vi "cam1 analyse.vi"() -> (0 "W3&color":string)   [LabVIEW 2019]
uses:
  <vilib>/vision/Classification.llb/IMAQ Classifier Read Options.ctl
  <vilib>/vision/NI_Vision_Development_Module.lvlib
panel:
  out "R9 chiffre":string
  out "R8 chiffre":string
  out "R6 chiffre":string
  out "R3 chiffre":string
  out "B9 chiffre":string
  out "B8 chiffre":string
  out "B7 chiffre":string
  out "B6 chiffre":string
  out "B4 chiffre":string
  out "B3 chiffre":string
  out "B2 chiffre":string
  out "B1 chiffre":string
  out "W4 chiffre":string
  out "W6 chiffre":string
  out "W1 chiffre":string
  out "W2 chiffre":string
  out "W3 chiffre":string
  in  "R9":T1={"Global Rectangle"=[0, 0, 1279, 959], "Contours"=[{"ID"=enum."External", "Type"=3, "Coordinates"=[0, 0, 1279, 959]}]} {"Contours"."Type" items=["No Selection", "Point", "Line", "Rectangle", "Oval", "Polygon", "Freehand Region", "Annulus", "Unused2", "Unused3", "Broken Line", "Freehand Line", "Rotated Rectangle"]}
  out "R9":string[](array[string])
  in  "R8":T1={"Global Rectangle"=[0, 0, 1279, 959], "Contours"=[{"ID"=enum."External", "Type"=3, "Coordinates"=[0, 0, 1279, 959]}]} {"Contours"."Type" items=["No Selection", "Point", "Line", "Rectangle", "Oval", "Polygon", "Freehand Region", "Annulus", "Unused2", "Unused3", "Broken Line", "Freehand Line", "Rotated Rectangle"]}
  out "R8":string[](array[string])
  in  "R6":T1={"Global Rectangle"=[0, 0, 1279, 959], "Contours"=[{"ID"=enum."External", "Type"=3, "Coordinates"=[0, 0, 1279, 959]}]} {"Contours"."Type" items=["No Selection", "Point", "Line", "Rectangle", "Oval", "Polygon", "Freehand Region", "Annulus", "Unused2", "Unused3", "Broken Line", "Freehand Line", "Rotated Rectangle"]}
  out "R6":string[](array[string])
  in  "R3":T1={"Global Rectangle"=[0, 0, 1279, 959], "Contours"=[{"ID"=enum."External", "Type"=3, "Coordinates"=[0, 0, 1279, 959]}]} {"Contours"."Type" items=["No Selection", "Point", "Line", "Rectangle", "Oval", "Polygon", "Freehand Region", "Annulus", "Unused2", "Unused3", "Broken Line", "Freehand Line", "Rotated Rectangle"]}
  out "R3":string[](array[string])
  in  "B9":T1={"Global Rectangle"=[0, 0, 1279, 959], "Contours"=[{"ID"=enum."External", "Type"=3, "Coordinates"=[0, 0, 1279, 959]}]} {"Contours"."Type" items=["No Selection", "Point", "Line", "Rectangle", "Oval", "Polygon", "Freehand Region", "Annulus", "Unused2", "Unused3", "Broken Line", "Freehand Line", "Rotated Rectangle"]}
  out "B9":string[](array[string])
  in  "B8":T1={"Global Rectangle"=[0, 0, 1279, 959], "Contours"=[{"ID"=enum."External", "Type"=3, "Coordinates"=[0, 0, 1279, 959]}]} {"Contours"."Type" items=["No Selection", "Point", "Line", "Rectangle", "Oval", "Polygon", "Freehand Region", "Annulus", "Unused2", "Unused3", "Broken Line", "Freehand Line", "Rotated Rectangle"]}
  out "B8":string[](array[string])
  in  "B7":T1={"Global Rectangle"=[0, 0, 1279, 959], "Contours"=[{"ID"=enum."External", "Type"=3, "Coordinates"=[0, 0, 1279, 959]}]} {"Contours"."Type" items=["No Selection", "Point", "Line", "Rectangle", "Oval", "Polygon", "Freehand Region", "Annulus", "Unused2", "Unused3", "Broken Line", "Freehand Line", "Rotated Rectangle"]}
  out "B7":string[](array[string])
  in  "B6":T1={"Global Rectangle"=[0, 0, 1279, 959], "Contours"=[{"ID"=enum."External", "Type"=3, "Coordinates"=[0, 0, 1279, 959]}]} {"Contours"."Type" items=["No Selection", "Point", "Line", "Rectangle", "Oval", "Polygon", "Freehand Region", "Annulus", "Unused2", "Unused3", "Broken Line", "Freehand Line", "Rotated Rectangle"]}
  out "B6":string[](array[string])
  in  "B4":T1={"Global Rectangle"=[0, 0, 1279, 959], "Contours"=[{"ID"=enum."External", "Type"=3, "Coordinates"=[0, 0, 1279, 959]}]} {"Contours"."Type" items=["No Selection", "Point", "Line", "Rectangle", "Oval", "Polygon", "Freehand Region", "Annulus", "Unused2", "Unused3", "Broken Line", "Freehand Line", "Rotated Rectangle"]}
  out "B4":string[](array[string])
  in  "B3":T1={"Global Rectangle"=[0, 0, 1279, 959], "Contours"=[{"ID"=enum."External", "Type"=3, "Coordinates"=[0, 0, 1279, 959]}]} {"Contours"."Type" items=["No Selection", "Point", "Line", "Rectangle", "Oval", "Polygon", "Freehand Region", "Annulus", "Unused2", "Unused3", "Broken Line", "Freehand Line", "Rotated Rectangle"]}
  out "B3":string[](array[string])
  in  "B2":T1={"Global Rectangle"=[0, 0, 1279, 959], "Contours"=[{"ID"=enum."External", "Type"=3, "Coordinates"=[0, 0, 1279, 959]}]} {"Contours"."Type" items=["No Selection", "Point", "Line", "Rectangle", "Oval", "Polygon", "Freehand Region", "Annulus", "Unused2", "Unused3", "Broken Line", "Freehand Line", "Rotated Rectangle"]}
  out "B2":string[](array[string])
  in  "B1":T1={"Global Rectangle"=[0, 0, 1279, 959], "Contours"=[{"ID"=enum."External", "Type"=3, "Coordinates"=[0, 0, 1279, 959]}]} {"Contours"."Type" items=["No Selection", "Point", "Line", "Rectangle", "Oval", "Polygon", "Freehand Region", "Annulus", "Unused2", "Unused3", "Broken Line", "Freehand Line", "Rotated Rectangle"]}
  out "B1":string[](array[string])
  in  "W4":T1={"Global Rectangle"=[0, 0, 1279, 959], "Contours"=[{"ID"=enum."External", "Type"=3, "Coordinates"=[0, 0, 1279, 959]}]} {"Contours"."Type" items=["No Selection", "Point", "Line", "Rectangle", "Oval", "Polygon", "Freehand Region", "Annulus", "Unused2", "Unused3", "Broken Line", "Freehand Line", "Rotated Rectangle"]}
  out "W4":string[](array[string])
  in  "W6":T1={"Global Rectangle"=[0, 0, 1279, 959], "Contours"=[{"ID"=enum."External", "Type"=3, "Coordinates"=[0, 0, 1279, 959]}]} {"Contours"."Type" items=["No Selection", "Point", "Line", "Rectangle", "Oval", "Polygon", "Freehand Region", "Annulus", "Unused2", "Unused3", "Broken Line", "Freehand Line", "Rotated Rectangle"]}
  out "W6":string[](array[string])
  in  "W1":T1={"Global Rectangle"=[0, 0, 1279, 959], "Contours"=[{"ID"=enum."External", "Type"=3, "Coordinates"=[0, 0, 1279, 959]}]} {"Contours"."Type" items=["No Selection", "Point", "Line", "Rectangle", "Oval", "Polygon", "Freehand Region", "Annulus", "Unused2", "Unused3", "Broken Line", "Freehand Line", "Rotated Rectangle"]}
  out "W1":string[](array[string])
  out "W2":errorcluster
  in  "W2":T1={"Global Rectangle"=[0, 0, 1279, 959], "Contours"=[{"ID"=enum."External", "Type"=3, "Coordinates"=[0, 0, 1279, 959]}]} {"Contours"."Type" items=["No Selection", "Point", "Line", "Rectangle", "Oval", "Polygon", "Freehand Region", "Annulus", "Unused2", "Unused3", "Broken Line", "Freehand Line", "Rotated Rectangle"]}
  out "W2":string[](array[string])
  out "Coordinates":i32[](array[numeric])
  in  "W3":T1={"Global Rectangle"=[0, 0, 1279, 959], "Contours"=[{"ID"=enum."External", "Type"=3, "Coordinates"=[0, 0, 1279, 959]}]} {"Contours"."Type" items=["No Selection", "Point", "Line", "Rectangle", "Oval", "Polygon", "Freehand Region", "Annulus", "Unused2", "Unused3", "Broken Line", "Freehand Line", "Rotated Rectangle"]}
  out "Image Out":T2(plugin-control)
  out "W3":errorcluster
  out "W3":string[](array[string])
  in  "error in":errorcluster
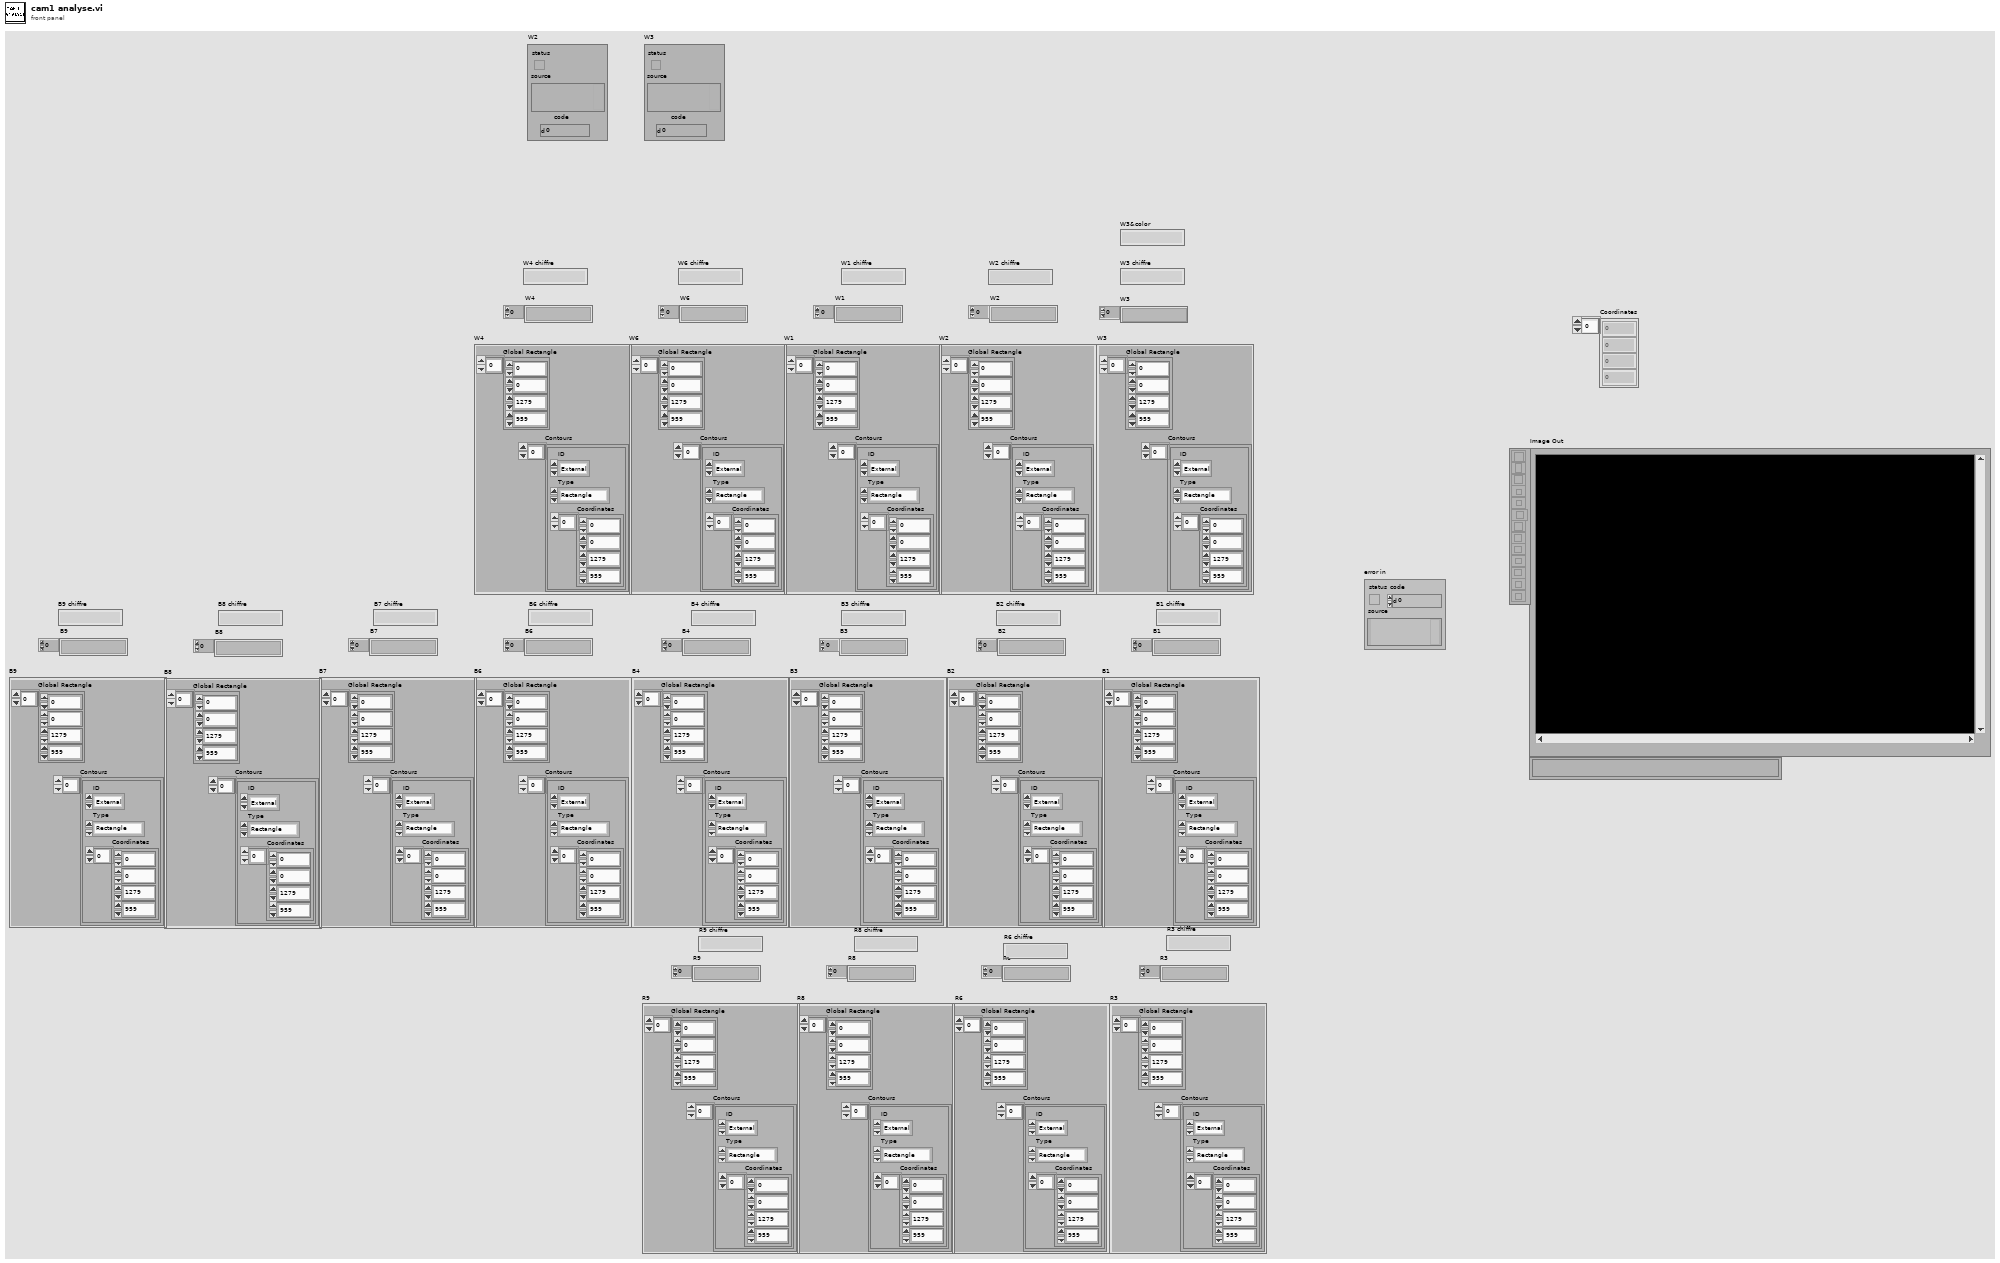
[diagram p1: front panel]
types:
  T1 = cluster{"Global Rectangle":i32[], "Contours":cluster{"ID":enum32{"External", "Internal"}, "Type":u32, "Coordinates":i32[]}[]}
  T2 = typedef "IMAQ Image.ctl" = refnum<image>
  T3 = typedef "IMAQ Classifier Read Options.ctl" = i32
  T4 = typedef "IMAQ Classifier Session.ctl" = refnum<k1>
  T5 = typedef "ROI Descriptor" = cluster{"Global Rectangle":i32[], "Contours":cluster{"ID":enum32{"External", "Internal"}, "Type":u32, "Coordinates":i32[]}[]}
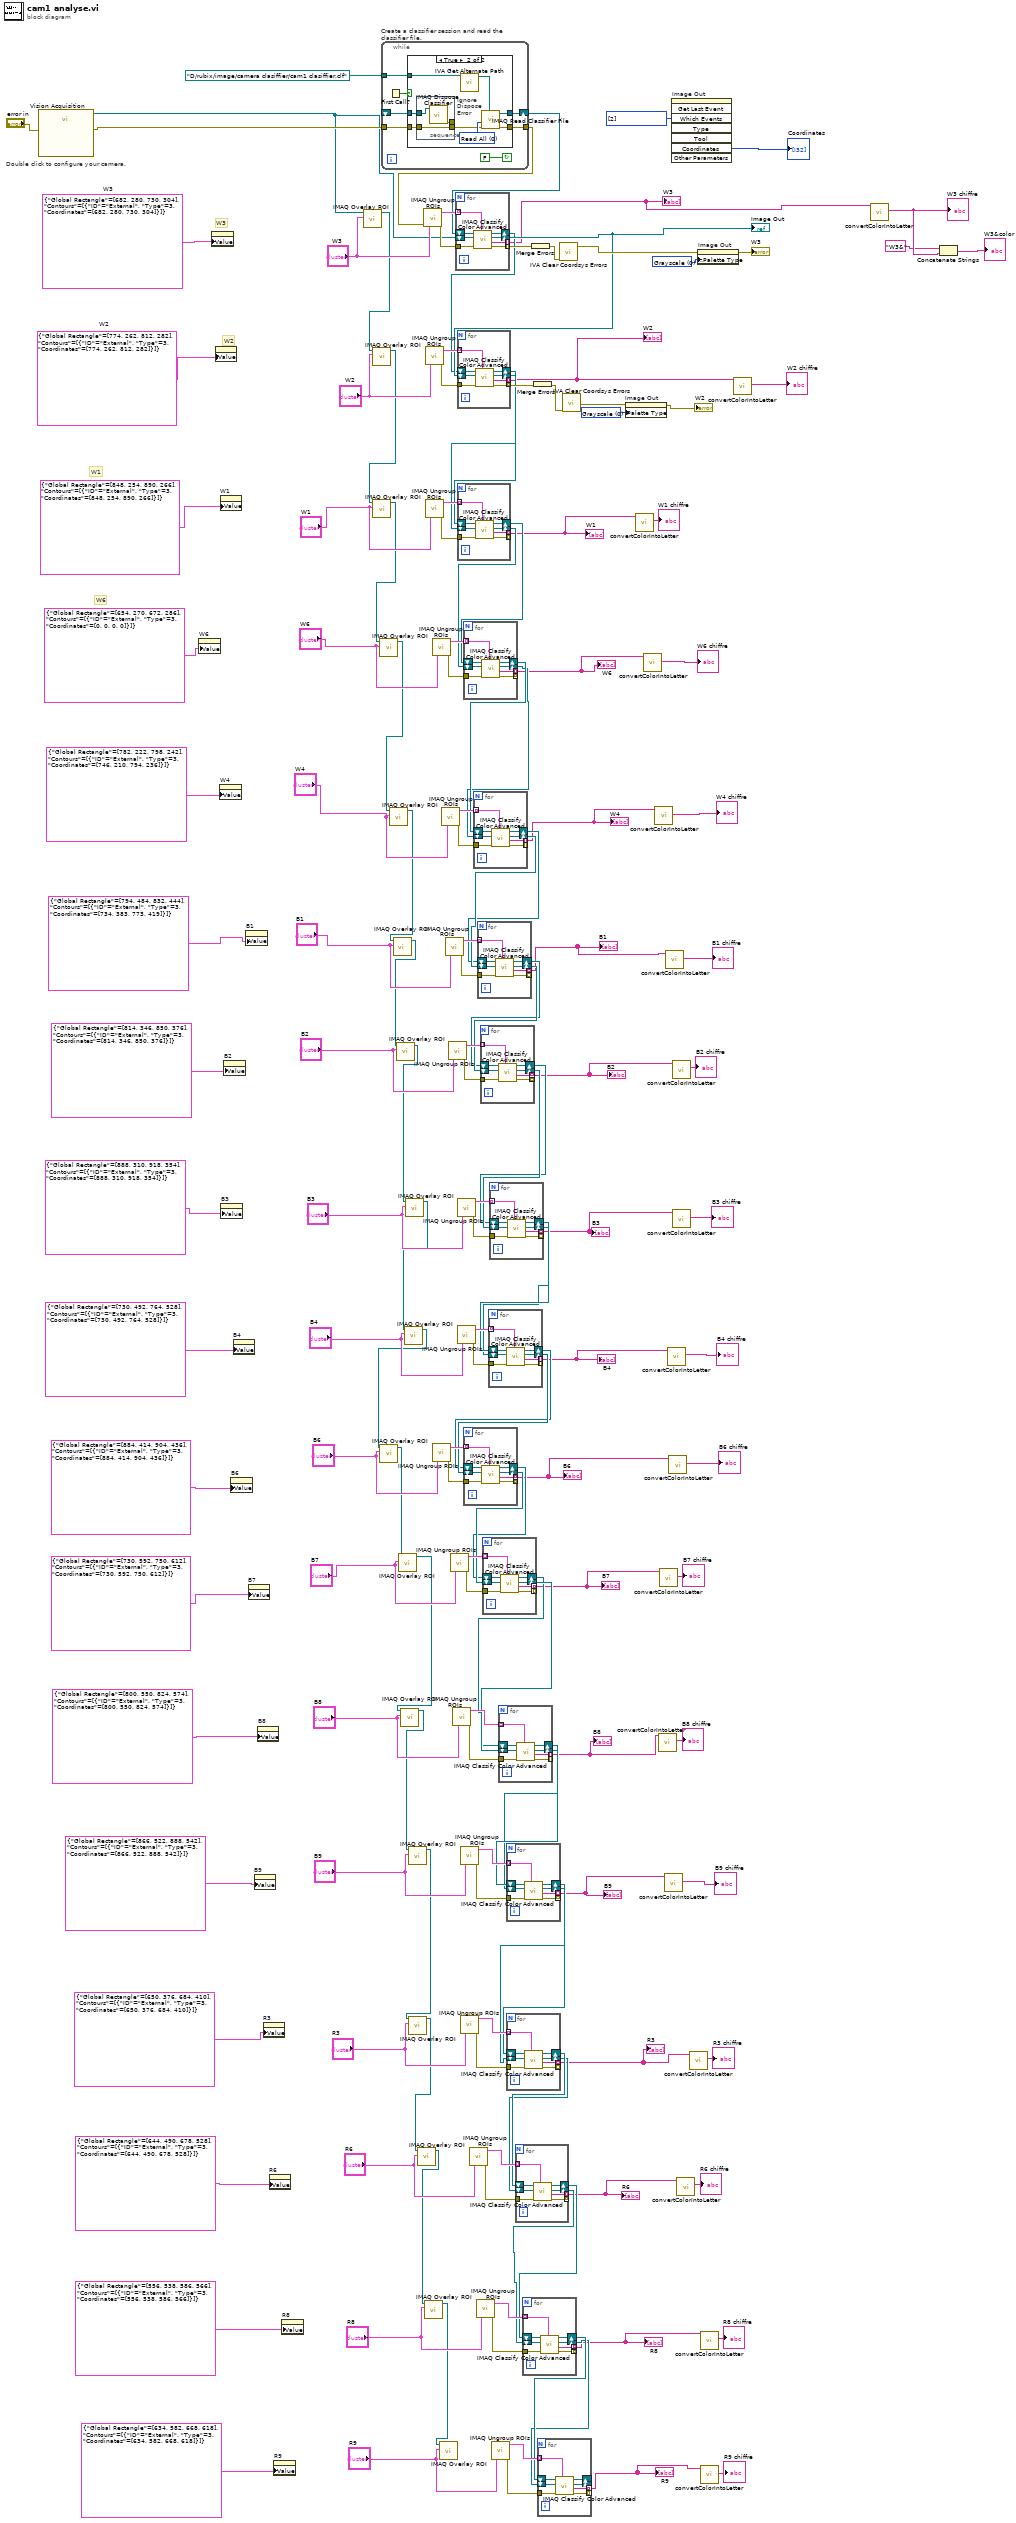
[diagram p0: block diagram]
diagram:
  w148 = u32 0 items=["Grayscale", "Binary", "Gradient", "Rainbow", "Temperature", "User Defined", "Binary 16 Bit", "Gradient 16 Bit", "Rainbow 16 Bit", "Temperature 16 Bit", "User Defined 16 Bit"] ("Palette:Palette Type")
  w158 = i32[] [2] items=["No Event"=0, "Click Event"=1, "Draw Event"=2, "Size Event"=4, "Scroll Event"=5, "Double Click Event"=8] ("Which Events")
  w159 = u32 0 items=["Grayscale", "Binary", "Gradient", "Rainbow", "Temperature", "User Defined", "Binary 16 Bit", "Gradient 16 Bit", "Rainbow 16 Bit", "Temperature 16 Bit", "User Defined 16 Bit"] ("Palette Type")
  # "W3"
  # "W2"
  # "W6"
  # "W1"
  # "Double click to configure your camera."
  n1 = call "Vision Acquisition"("error in"="error in") -> ("Image Out"=w144:T2, "error out"=w169:errorcluster)  [unwired: 24 in, 1 out]
  n2 = property on="W6" class="Clust (strict)"("Value"=T1 {"Global Rectangle"=[654, 270, 672, 286], "Contours"=[{"ID"=enum."External", "Type"=3, "Coordinates"=[0, 0, 0, 0]}]} ("ROI Descriptor (Color Classification 1)")) -> ()  [unwired: 2 in, 2 out]
  n3 = property on="W3" class="Clust (strict)"("Value"=T1 {"Global Rectangle"=[682, 280, 730, 304], "Contours"=[{"ID"=enum."External", "Type"=3, "Coordinates"=[682, 280, 730, 304]}]} ("ROI Descriptor (Color Classification 1)")) -> ()  [unwired: 2 in, 2 out]
  n4 = property on="W2" class="Clust (strict)"("Value"=T1 {"Global Rectangle"=[774, 262, 812, 282], "Contours"=[{"ID"=enum."External", "Type"=3, "Coordinates"=[774, 262, 812, 282]}]} ("ROI Descriptor (Color Classification 1)")) -> ()  [unwired: 2 in, 2 out]
  n5 = property on="W4" class="Clust (strict)"("Value"=T1 {"Global Rectangle"=[782, 222, 798, 242], "Contours"=[{"ID"=enum."External", "Type"=3, "Coordinates"=[746, 210, 794, 236]}]} ("ROI Descriptor (Color Classification 1)")) -> ()  [unwired: 2 in, 2 out]
  n6 = property on="W1" class="Clust (strict)"("Value"=T1 {"Global Rectangle"=[848, 254, 890, 266], "Contours"=[{"ID"=enum."External", "Type"=3, "Coordinates"=[848, 254, 890, 266]}]} ("ROI Descriptor (Color Classification 1)")) -> ()  [unwired: 2 in, 2 out]
  n7 = property on="B3" class="Clust (strict)"("Value"=T1 {"Global Rectangle"=[888, 310, 918, 354], "Contours"=[{"ID"=enum."External", "Type"=3, "Coordinates"=[888, 310, 918, 354]}]} ("ROI Descriptor (Color Classification 1)")) -> ()  [unwired: 2 in, 2 out]
  n8 = property on="B2" class="Clust (strict)"("Value"=T1 {"Global Rectangle"=[814, 346, 850, 376], "Contours"=[{"ID"=enum."External", "Type"=3, "Coordinates"=[814, 346, 850, 376]}]} ("ROI Descriptor (Color Classification 1)")) -> ()  [unwired: 2 in, 2 out]
  n9 = property on="B6" class="Clust (strict)"("Value"=T1 {"Global Rectangle"=[884, 414, 904, 436], "Contours"=[{"ID"=enum."External", "Type"=3, "Coordinates"=[884, 414, 904, 436]}]} ("ROI Descriptor (Color Classification 1)")) -> ()  [unwired: 2 in, 2 out]
  n10 = property on="B4" class="Clust (strict)"("Value"=T1 {"Global Rectangle"=[730, 492, 764, 528], "Contours"=[{"ID"=enum."External", "Type"=3, "Coordinates"=[730, 492, 764, 528]}]} ("ROI Descriptor (Color Classification 1)")) -> ()  [unwired: 2 in, 2 out]
  n11 = property on="B1" class="Clust (strict)"("Value"=T1 {"Global Rectangle"=[794, 484, 832, 444], "Contours"=[{"ID"=enum."External", "Type"=3, "Coordinates"=[734, 383, 773, 419]}]} ("ROI Descriptor (Color Classification 1)")) -> ()  [unwired: 2 in, 2 out]
  n12 = property on="B7" class="Clust (strict)"("Value"=T1 {"Global Rectangle"=[730, 592, 750, 612], "Contours"=[{"ID"=enum."External", "Type"=3, "Coordinates"=[730, 592, 750, 612]}]} ("ROI Descriptor (Color Classification 1)")) -> ()  [unwired: 2 in, 2 out]
  n13 = property on="B9" class="Clust (strict)"("Value"=T1 {"Global Rectangle"=[866, 522, 888, 542], "Contours"=[{"ID"=enum."External", "Type"=3, "Coordinates"=[866, 522, 888, 542]}]} ("ROI Descriptor (Color Classification 1)")) -> ()  [unwired: 2 in, 2 out]
  n14 = property on="B8" class="Clust (strict)"("Value"=T1 {"Global Rectangle"=[800, 550, 824, 574], "Contours"=[{"ID"=enum."External", "Type"=3, "Coordinates"=[800, 550, 824, 574]}]} ("ROI Descriptor (Color Classification 1)")) -> ()  [unwired: 2 in, 2 out]
  n15 = property on="R3" class="Clust (strict)"("Value"=T1 {"Global Rectangle"=[650, 376, 684, 410], "Contours"=[{"ID"=enum."External", "Type"=3, "Coordinates"=[650, 376, 684, 410]}]} ("ROI Descriptor (Color Classification 1)")) -> ()  [unwired: 2 in, 2 out]
  n16 = property on="R6" class="Clust (strict)"("Value"=T1 {"Global Rectangle"=[644, 490, 678, 528], "Contours"=[{"ID"=enum."External", "Type"=3, "Coordinates"=[644, 490, 678, 528]}]} ("ROI Descriptor (Color Classification 1)")) -> ()  [unwired: 2 in, 2 out]
  n17 = property on="R9" class="Clust (strict)"("Value"=T1 {"Global Rectangle"=[634, 582, 668, 618], "Contours"=[{"ID"=enum."External", "Type"=3, "Coordinates"=[634, 582, 668, 618]}]} ("ROI Descriptor (Color Classification 1)")) -> ()  [unwired: 2 in, 2 out]
  n18 = property on="R8" class="Clust (strict)"("Value"=T1 {"Global Rectangle"=[556, 538, 586, 566], "Contours"=[{"ID"=enum."External", "Type"=3, "Coordinates"=[556, 538, 586, 566]}]} ("ROI Descriptor (Color Classification 1)")) -> ()  [unwired: 2 in, 2 out]
  n19 = call "IMAQ Overlay ROI"("ROI Descriptor"="W3", "Image"=w144) -> ("Image Out"=w146:T2)  [unwired: 8 in, 1 out]
  n20 = call "IMAQ Overlay ROI"("ROI Descriptor"="W2", "Image"=w146) -> ("Image Out"=w139:T2)  [unwired: 8 in, 1 out]
  n21 = call "IMAQ Overlay ROI"("ROI Descriptor"="W1", "Image"=w139) -> ("Image Out"=w131:T2)  [unwired: 8 in, 1 out]
  n22 = call "IMAQ Overlay ROI"("ROI Descriptor"="W6", "Image"=w131) -> ("Image Out"=w123:T2)  [unwired: 8 in, 1 out]
  n23 = while "Create a classifier session and read the classifier file." {
    shift-right: [w177] -> w161
    shift-left: _ -> [w176]
    tunnel: w169 -> [w174]
    tunnel: [w173] -> w167
    tunnel: path "D:/rubix/image/camera clasiffier/cam1 clasiffier.clf" ("File Path") -> [w172]
    stop <- FALSE continue-if-true
    n24 = First Call?() -> (First Call?: T/F=w171:bool)
    n25 = case shown="True" w171 {
      tunnel: [w179 w186] -> w177
      tunnel: w176 -> [w179 w184]
      tunnel: w174 -> [w178 w183]
      tunnel: [w178 w185] -> w173
      tunnel: w172 -> [_ w181]
      frame False {
      }
      frame True {
        w187 = T3 0 items=["Read All", "Add Samples, Do Not Change Options", "Read Options, Do Not Add Samples"] ("Read Options")
        # "Ignore Dispose Error"
        n26 = stacked-sequence {
          tunnel: w184 -> [w190]
          tunnel: w183 -> [w189]
          tunnel: [w189] -> w182
          tunnel: [w188] -> _
          frame #0 {
            n27 = call "IMAQ Dispose Classifier"("Classifier Session"=w190) -> ("error out"=w188:errorcluster)  [unwired: 1 in, 9 out]
          }
        }
        n28 = call <vilib>:"IVA Get Alternate Path.vi"("Path In"=w181) -> ("Path Out"=w180:path)  [unwired: 10 out]
        n29 = call "IMAQ Read Classifier File"("File Path"=w180, "error in (no error)"=w182, "Read Options"=w187) -> ("error out"=w185:errorcluster, "Classifier Session"=w186:T4)  [unwired: 1 in, 6 out]
      }
    }
  }
  n30 = call "IMAQ Overlay ROI"("ROI Descriptor"="W4", "Image"=w123) -> ("Image Out"=w116:T2)  [unwired: 8 in, 1 out]
  n31 = call "IMAQ Overlay ROI"("ROI Descriptor"="B1", "Image"=w116) -> ("Image Out"=w111:T2)  [unwired: 8 in, 1 out]
  n32 = call "IMAQ Overlay ROI"("ROI Descriptor"="B2", "Image"=w111) -> ("Image Out"=w104:T2)  [unwired: 8 in, 1 out]
  n33 = call "IMAQ Overlay ROI"("ROI Descriptor"="B3", "Image"=w104) -> ("Image Out"=w94:T2)  [unwired: 8 in, 1 out]
  n34 = call "IMAQ Overlay ROI"("ROI Descriptor"="B4", "Image"=w94) -> ("Image Out"=w90:T2)  [unwired: 8 in, 1 out]
  n35 = call "IMAQ Overlay ROI"("ROI Descriptor"="B6", "Image"=w90) -> ("Image Out"=w81:T2)  [unwired: 8 in, 1 out]
  n36 = call "IMAQ Overlay ROI"("ROI Descriptor"="B7", "Image"=w81) -> ("Image Out"=w76:T2)  [unwired: 8 in, 1 out]
  n37 = call "IMAQ Overlay ROI"("ROI Descriptor"="B8", "Image"=w76) -> ("Image Out"=w69:T2)  [unwired: 8 in, 1 out]
  n38 = call "IMAQ Overlay ROI"("ROI Descriptor"="B9", "Image"=w69) -> ("Image Out"=w62:T2)  [unwired: 8 in, 1 out]
  n39 = call "IMAQ Overlay ROI"("ROI Descriptor"="R3", "Image"=w62) -> ("Image Out"=w55:T2)  [unwired: 8 in, 1 out]
  n40 = call "IMAQ Overlay ROI"("ROI Descriptor"="R6", "Image"=w55) -> ("Image Out"=w48:T2)  [unwired: 8 in, 1 out]
  n41 = call "IMAQ Ungroup ROIs"("error in (no error)"=w167, "ROI Descriptor"="W3") -> ("error out"=w166:errorcluster, "ROI Descriptors out"=w165:T5[])  [unwired: 2 out]
  n42 = call "IMAQ Overlay ROI"("ROI Descriptor"="R8", "Image"=w48) -> ("Image Out"=w41:T2)  [unwired: 8 in, 1 out]
  n43 = call "IMAQ Ungroup ROIs"("ROI Descriptor"="W2") -> ("error out"=w154:errorcluster, "ROI Descriptors out"=w153:T5[])  [unwired: 1 in, 2 out]
  n44 = call "IMAQ Ungroup ROIs"("ROI Descriptor"="W1") -> ("error out"=w141:errorcluster, "ROI Descriptors out"=w140:T5[])  [unwired: 1 in, 2 out]
  n45 = call "IMAQ Ungroup ROIs"("ROI Descriptor"="W6") -> ("error out"=w134:errorcluster, "ROI Descriptors out"=w133:T5[])  [unwired: 1 in, 2 out]
  n46 = call "IMAQ Ungroup ROIs"("ROI Descriptor"="B6") -> ("error out"=w93:errorcluster, "ROI Descriptors out"=w92:T5[])  [unwired: 1 in, 2 out]
  n47 = call "IMAQ Overlay ROI"("ROI Descriptor"="R9", "Image"=w41) -> ()  [unwired: 8 in, 2 out]
  n48 = call "IMAQ Ungroup ROIs"("ROI Descriptor"="W4") -> ("error out"=w127:errorcluster, "ROI Descriptors out"=w126:T5[])  [unwired: 1 in, 2 out]
  n49 = call "IMAQ Ungroup ROIs"("ROI Descriptor"="B1") -> ("error out"=w120:errorcluster, "ROI Descriptors out"=w119:T5[])  [unwired: 1 in, 2 out]
  n50 = call "IMAQ Ungroup ROIs"("ROI Descriptor"="B2") -> ("error out"=w114:errorcluster, "ROI Descriptors out"=w113:T5[])  [unwired: 1 in, 2 out]
  n51 = call "IMAQ Ungroup ROIs"("ROI Descriptor"="B7") -> ("error out"=w86:errorcluster, "ROI Descriptors out"=w85:T5[])  [unwired: 1 in, 2 out]
  n52 = call "IMAQ Ungroup ROIs"("ROI Descriptor"="B8") -> ("error out"=w79:errorcluster, "ROI Descriptors out"=w78:T5[])  [unwired: 1 in, 2 out]
  n53 = for {
    tunnel: [w198] -> w20 mode=indexing
    tunnel: [w197] -> w164 mode=indexing
    tunnel: w166 -> [w195]
    tunnel: w165 -> [w194] mode=indexing
    shift-right: [w192] -> w143
    shift-left: w144 -> [w193]
    shift-right: [w191] -> w142
    shift-left: w161 -> [w196]
    n54 = call "IMAQ Classify Color Advanced"("ROI Descriptor"=w194, "error in (no error)"=w195, "Image"=w193, "Classifier Session"=w196) -> ("error out"=w197:errorcluster, "Class"=w198:string, "Image (dup)"=w192:T2, "Classifier Session (dup)"=w191:T4)  [unwired: 4 out]
  }
  "W3" <- w20
  "Image Out" <- w143
  n55 = for {
    tunnel: [w206] -> w36 mode=indexing
    tunnel: [w205] -> w152 mode=indexing
    tunnel: w154 -> [w203]
    tunnel: w153 -> [w202] mode=indexing
    shift-right: [w200] -> w137
    shift-left: w143 -> [w201]
    shift-right: [w199] -> w138
    shift-left: w142 -> [w204]
    n56 = call "IMAQ Classify Color Advanced"("ROI Descriptor"=w202, "error in (no error)"=w203, "Image"=w201, "Classifier Session"=w204) -> ("error out"=w205:errorcluster, "Class"=w206:string, "Image (dup)"=w200:T2, "Classifier Session (dup)"=w199:T4)  [unwired: 4 out]
  }
  "W2" <- w36
  n57 = for {
    tunnel: [w214] -> w35 mode=indexing
    tunnel: [w213] -> _ mode=indexing
    tunnel: w141 -> [w211]
    tunnel: w140 -> [w210] mode=indexing
    shift-right: [w208] -> w130
    shift-left: w137 -> [w209]
    shift-right: [w207] -> w129
    shift-left: w138 -> [w212]
    n58 = call "IMAQ Classify Color Advanced"("ROI Descriptor"=w210, "error in (no error)"=w211, "Image"=w209, "Classifier Session"=w212) -> ("error out"=w213:errorcluster, "Class"=w214:string, "Image (dup)"=w208:T2, "Classifier Session (dup)"=w207:T4)  [unwired: 4 out]
  }
  "W1" <- w35
  n59 = call "IMAQ Ungroup ROIs"("ROI Descriptor"="B4") -> ("error out"=w100:errorcluster, "ROI Descriptors out"=w99:T5[])  [unwired: 1 in, 2 out]
  n60 = call "IMAQ Ungroup ROIs"("ROI Descriptor"="B3") -> ("error out"=w107:errorcluster, "ROI Descriptors out"=w106:T5[])  [unwired: 1 in, 2 out]
  n61 = call "IMAQ Ungroup ROIs"("ROI Descriptor"="B9") -> ("error out"=w72:errorcluster, "ROI Descriptors out"=w71:T5[])  [unwired: 1 in, 2 out]
  n62 = call "IMAQ Ungroup ROIs"("ROI Descriptor"="R3") -> ("error out"=w65:errorcluster, "ROI Descriptors out"=w64:T5[])  [unwired: 1 in, 2 out]
  n63 = for {
    tunnel: [w222] -> w34 mode=indexing
    tunnel: [w221] -> _ mode=indexing
    tunnel: w134 -> [w219]
    tunnel: w133 -> [w218] mode=indexing
    shift-right: [w216] -> w124
    shift-left: w130 -> [w217]
    shift-right: [w215] -> w125
    shift-left: w129 -> [w220]
    n64 = call "IMAQ Classify Color Advanced"("ROI Descriptor"=w218, "error in (no error)"=w219, "Image"=w217, "Classifier Session"=w220) -> ("error out"=w221:errorcluster, "Class"=w222:string, "Image (dup)"=w216:T2, "Classifier Session (dup)"=w215:T4)  [unwired: 4 out]
  }
  "W6" <- w34
  n65 = call "IMAQ Ungroup ROIs"("ROI Descriptor"="R6") -> ("error out"=w58:errorcluster, "ROI Descriptors out"=w57:T5[])  [unwired: 1 in, 2 out]
  n66 = for {
    tunnel: [w230] -> w33 mode=indexing
    tunnel: [w229] -> _ mode=indexing
    tunnel: w127 -> [w227]
    tunnel: w126 -> [w226] mode=indexing
    shift-right: [w224] -> w118
    shift-left: w124 -> [w225]
    shift-right: [w223] -> w117
    shift-left: w125 -> [w228]
    n67 = call "IMAQ Classify Color Advanced"("ROI Descriptor"=w226, "error in (no error)"=w227, "Image"=w225, "Classifier Session"=w228) -> ("error out"=w229:errorcluster, "Class"=w230:string, "Image (dup)"=w224:T2, "Classifier Session (dup)"=w223:T4)  [unwired: 4 out]
  }
  "W4" <- w33
  n68 = call "IMAQ Ungroup ROIs"("ROI Descriptor"="R8") -> ("error out"=w51:errorcluster, "ROI Descriptors out"=w50:T5[])  [unwired: 1 in, 2 out]
  n69 = for {
    tunnel: [w238] -> w32 mode=indexing
    tunnel: [w237] -> _ mode=indexing
    tunnel: w120 -> [w235]
    tunnel: w119 -> [w234] mode=indexing
    shift-right: [w232] -> w110
    shift-left: w118 -> [w233]
    shift-right: [w231] -> w109
    shift-left: w117 -> [w236]
    n70 = call "IMAQ Classify Color Advanced"("ROI Descriptor"=w234, "error in (no error)"=w235, "Image"=w233, "Classifier Session"=w236) -> ("error out"=w237:errorcluster, "Class"=w238:string, "Image (dup)"=w232:T2, "Classifier Session (dup)"=w231:T4)  [unwired: 4 out]
  }
  "B1" <- w32
  n71 = for {
    tunnel: [w246] -> w31 mode=indexing
    tunnel: [w245] -> _ mode=indexing
    tunnel: w114 -> [w243]
    tunnel: w113 -> [w242] mode=indexing
    shift-right: [w240] -> w103
    shift-left: w110 -> [w241]
    shift-right: [w239] -> w102
    shift-left: w109 -> [w244]
    n72 = call "IMAQ Classify Color Advanced"("ROI Descriptor"=w242, "error in (no error)"=w243, "Image"=w241, "Classifier Session"=w244) -> ("error out"=w245:errorcluster, "Class"=w246:string, "Image (dup)"=w240:T2, "Classifier Session (dup)"=w239:T4)  [unwired: 4 out]
  }
  "B2" <- w31
  n73 = for {
    tunnel: [w254] -> w30 mode=indexing
    tunnel: [w253] -> _ mode=indexing
    tunnel: w107 -> [w251]
    tunnel: w106 -> [w250] mode=indexing
    shift-right: [w248] -> w97
    shift-left: w103 -> [w249]
    shift-right: [w247] -> w98
    shift-left: w102 -> [w252]
    n74 = call "IMAQ Classify Color Advanced"("ROI Descriptor"=w250, "error in (no error)"=w251, "Image"=w249, "Classifier Session"=w252) -> ("error out"=w253:errorcluster, "Class"=w254:string, "Image (dup)"=w248:T2, "Classifier Session (dup)"=w247:T4)  [unwired: 4 out]
  }
  "B3" <- w30
  n75 = for {
    tunnel: [w262] -> w29 mode=indexing
    tunnel: [w261] -> _ mode=indexing
    tunnel: w100 -> [w259]
    tunnel: w99 -> [w258] mode=indexing
    shift-right: [w256] -> w89
    shift-left: w97 -> [w257]
    shift-right: [w255] -> w88
    shift-left: w98 -> [w260]
    n76 = call "IMAQ Classify Color Advanced"("ROI Descriptor"=w258, "error in (no error)"=w259, "Image"=w257, "Classifier Session"=w260) -> ("error out"=w261:errorcluster, "Class"=w262:string, "Image (dup)"=w256:T2, "Classifier Session (dup)"=w255:T4)  [unwired: 4 out]
  }
  "B4" <- w29
  n77 = for {
    tunnel: [w270] -> w28 mode=indexing
    tunnel: [w269] -> _ mode=indexing
    tunnel: w93 -> [w267]
    tunnel: w92 -> [w266] mode=indexing
    shift-right: [w264] -> w84
    shift-left: w89 -> [w265]
    shift-right: [w263] -> w83
    shift-left: w88 -> [w268]
    n78 = call "IMAQ Classify Color Advanced"("ROI Descriptor"=w266, "error in (no error)"=w267, "Image"=w265, "Classifier Session"=w268) -> ("error out"=w269:errorcluster, "Class"=w270:string, "Image (dup)"=w264:T2, "Classifier Session (dup)"=w263:T4)  [unwired: 4 out]
  }
  "B6" <- w28
  n79 = for {
    tunnel: [w278] -> w27 mode=indexing
    tunnel: [w277] -> _ mode=indexing
    tunnel: w86 -> [w275]
    tunnel: w85 -> [w274] mode=indexing
    shift-right: [w272] -> w75
    shift-left: w84 -> [w273]
    shift-right: [w271] -> w74
    shift-left: w83 -> [w276]
    n80 = call "IMAQ Classify Color Advanced"("ROI Descriptor"=w274, "error in (no error)"=w275, "Image"=w273, "Classifier Session"=w276) -> ("error out"=w277:errorcluster, "Class"=w278:string, "Image (dup)"=w272:T2, "Classifier Session (dup)"=w271:T4)  [unwired: 4 out]
  }
  "B7" <- w27
  n81 = call "IMAQ Ungroup ROIs"("ROI Descriptor"="R9") -> ("error out"=w44:errorcluster, "ROI Descriptors out"=w43:T5[])  [unwired: 1 in, 2 out]
  n82 = for {
    tunnel: [w286] -> w26 mode=indexing
    tunnel: [w285] -> _ mode=indexing
    tunnel: w79 -> [w283]
    tunnel: w78 -> [w282] mode=indexing
    shift-right: [w280] -> w67
    shift-left: w75 -> [w281]
    shift-right: [w279] -> w68
    shift-left: w74 -> [w284]
    n83 = call "IMAQ Classify Color Advanced"("ROI Descriptor"=w282, "error in (no error)"=w283, "Image"=w281, "Classifier Session"=w284) -> ("error out"=w285:errorcluster, "Class"=w286:string, "Image (dup)"=w280:T2, "Classifier Session (dup)"=w279:T4)  [unwired: 4 out]
  }
  "B8" <- w26
  n84 = for {
    tunnel: [w294] -> w25 mode=indexing
    tunnel: [w293] -> _ mode=indexing
    tunnel: w72 -> [w291]
    tunnel: w71 -> [w290] mode=indexing
    shift-right: [w288] -> w60
    shift-left: w67 -> [w289]
    shift-right: [w287] -> w61
    shift-left: w68 -> [w292]
    n85 = call "IMAQ Classify Color Advanced"("ROI Descriptor"=w290, "error in (no error)"=w291, "Image"=w289, "Classifier Session"=w292) -> ("error out"=w293:errorcluster, "Class"=w294:string, "Image (dup)"=w288:T2, "Classifier Session (dup)"=w287:T4)  [unwired: 4 out]
  }
  "B9" <- w25
  n86 = for {
    tunnel: [w302] -> w24 mode=indexing
    tunnel: [w301] -> _ mode=indexing
    tunnel: w65 -> [w299]
    tunnel: w64 -> [w298] mode=indexing
    shift-right: [w296] -> w53
    shift-left: w60 -> [w297]
    shift-right: [w295] -> w54
    shift-left: w61 -> [w300]
    n87 = call "IMAQ Classify Color Advanced"("ROI Descriptor"=w298, "error in (no error)"=w299, "Image"=w297, "Classifier Session"=w300) -> ("error out"=w301:errorcluster, "Class"=w302:string, "Image (dup)"=w296:T2, "Classifier Session (dup)"=w295:T4)  [unwired: 4 out]
  }
  "R3" <- w24
  n88 = for {
    tunnel: [w310] -> w23 mode=indexing
    tunnel: [w309] -> _ mode=indexing
    tunnel: w58 -> [w307]
    tunnel: w57 -> [w306] mode=indexing
    shift-right: [w304] -> w47
    shift-left: w53 -> [w305]
    shift-right: [w303] -> w46
    shift-left: w54 -> [w308]
    n89 = call "IMAQ Classify Color Advanced"("ROI Descriptor"=w306, "error in (no error)"=w307, "Image"=w305, "Classifier Session"=w308) -> ("error out"=w309:errorcluster, "Class"=w310:string, "Image (dup)"=w304:T2, "Classifier Session (dup)"=w303:T4)  [unwired: 4 out]
  }
  "R6" <- w23
  n90 = for {
    tunnel: [w318] -> w22 mode=indexing
    tunnel: [w317] -> _ mode=indexing
    tunnel: w51 -> [w315]
    tunnel: w50 -> [w314] mode=indexing
    shift-right: [w312] -> w39
    shift-left: w47 -> [w313]
    shift-right: [w311] -> w40
    shift-left: w46 -> [w316]
    n91 = call "IMAQ Classify Color Advanced"("ROI Descriptor"=w314, "error in (no error)"=w315, "Image"=w313, "Classifier Session"=w316) -> ("error out"=w317:errorcluster, "Class"=w318:string, "Image (dup)"=w312:T2, "Classifier Session (dup)"=w311:T4)  [unwired: 4 out]
  }
  "R8" <- w22
  n92 = Merge Errors(w164) -> (w163:errorcluster)
  n93 = Merge Errors(w152) -> (w151:errorcluster)
  n94 = for {
    tunnel: [w326] -> w21 mode=indexing
    tunnel: [w325] -> _ mode=indexing
    tunnel: w44 -> [w323]
    tunnel: w43 -> [w322] mode=indexing
    shift-right: [w320] -> _
    shift-left: w39 -> [w321]
    shift-right: [w319] -> _
    shift-left: w40 -> [w324]
    n95 = call "IMAQ Classify Color Advanced"("ROI Descriptor"=w322, "error in (no error)"=w323, "Image"=w321, "Classifier Session"=w324) -> ("error out"=w325:errorcluster, "Class"=w326:string, "Image (dup)"=w320:T2, "Classifier Session (dup)"=w319:T4)  [unwired: 4 out]
  }
  "R9" <- w21
  n96 = call <vilib>:"IVA Clear Coordsys Errors.vi"("error in (no error)"=w163) -> ("error out"=w162:errorcluster)  [unwired: 10 in]
  n97 = call <vilib>:"IVA Clear Coordsys Errors.vi"("error in (no error)"=w151) -> ("error out"=w149:errorcluster)  [unwired: 10 in]
  n98 = property on="Image Out" class="ImageControl"(error in=w149, "Palette Type"=w148) -> (error out=→"W2":errorcluster)  [unwired: 1 in, 1 out]
  n99 = call "convertColorIntoLetter.vi"("Array"=w35) -> ("String"=→"W1 chiffre":string)  [unwired: 10 in]
  n100 = call "convertColorIntoLetter.vi"("Array"=w34) -> ("String"=→"W6 chiffre":string)  [unwired: 10 in]
  n101 = call "convertColorIntoLetter.vi"("Array"=w33) -> ("String"=→"W4 chiffre":string)  [unwired: 10 in]
  n102 = call "convertColorIntoLetter.vi"("Array"=w26) -> ("String"=→"B8 chiffre":string)  [unwired: 10 in]
  n103 = call "convertColorIntoLetter.vi"("Array"=w27) -> ("String"=→"B7 chiffre":string)  [unwired: 10 in]
  n104 = call "convertColorIntoLetter.vi"("Array"=w25) -> ("String"=→"B9 chiffre":string)  [unwired: 10 in]
  n105 = call "convertColorIntoLetter.vi"("Array"=w32) -> ("String"=→"B1 chiffre":string)  [unwired: 10 in]
  n106 = call "convertColorIntoLetter.vi"("Array"=w29) -> ("String"=→"B4 chiffre":string)  [unwired: 10 in]
  n107 = call "convertColorIntoLetter.vi"("Array"=w28) -> ("String"=→"B6 chiffre":string)  [unwired: 10 in]
  n108 = invoke on="Image Out" class="ImageControl" method="Get Last Event"("Which Events"=w158) -> ("Coordinates"=→"Coordinates":i32[])  [unwired: 7 in, 7 out]
  n109 = call "convertColorIntoLetter.vi"("Array"=w31) -> ("String"=→"B2 chiffre":string)  [unwired: 10 in]
  n110 = call "convertColorIntoLetter.vi"("Array"=w30) -> ("String"=→"B3 chiffre":string)  [unwired: 10 in]
  n111 = call "convertColorIntoLetter.vi"("Array"=w23) -> ("String"=→"R6 chiffre":string)  [unwired: 10 in]
  n112 = call "convertColorIntoLetter.vi"("Array"=w24) -> ("String"=→"R3 chiffre":string)  [unwired: 10 in]
  n113 = property on="Image Out" class="ImageControl"(error in=w162, "Palette:Palette Type"=w159) -> (error out=→"W3":errorcluster)  [unwired: 1 in, 1 out]
  n114 = call "convertColorIntoLetter.vi"("Array"=w22) -> ("String"=→"R8 chiffre":string)  [unwired: 10 in]
  n115 = call "convertColorIntoLetter.vi"("Array"=w21) -> ("String"=→"R9 chiffre":string)  [unwired: 10 in]
  n116 = call "convertColorIntoLetter.vi"("Array"=w36) -> ("String"=→"W2 chiffre":string)  [unwired: 10 in]
  n117 = call "convertColorIntoLetter.vi"("Array"=w20) -> ("String"=w2:string)  [unwired: 10 in]
  "W3 chiffre" <- w2
  n118 = Concatenate Strings("W3&" ("string"), w2) -> (→"W3&color":string)
